vi "Nicmos_Diagnostics.vi"() -> ()   [LabVIEW 2009]
panel:
  in  "Difference:":bool
  out "Waveform at Coord":dbl[](graph)
  out "Intensity Map At Index":dbl[][](graph)
  in  "stop":bool
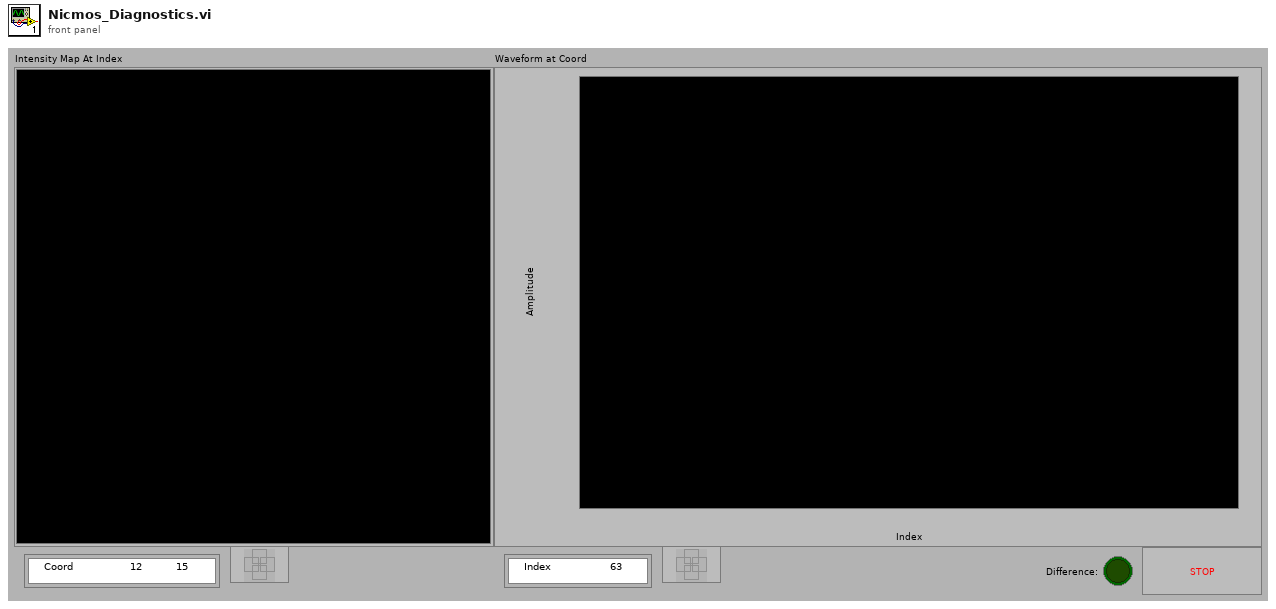
[diagram p1: front panel]
types:
  T1 = typedef "LVPointDoubleTypeDef.ctl" = cluster{"Cursor X":dbl, "Cursor Y":dbl}
  T2 = typedef "NICMOS.RAW.ctl" = u16[][][]
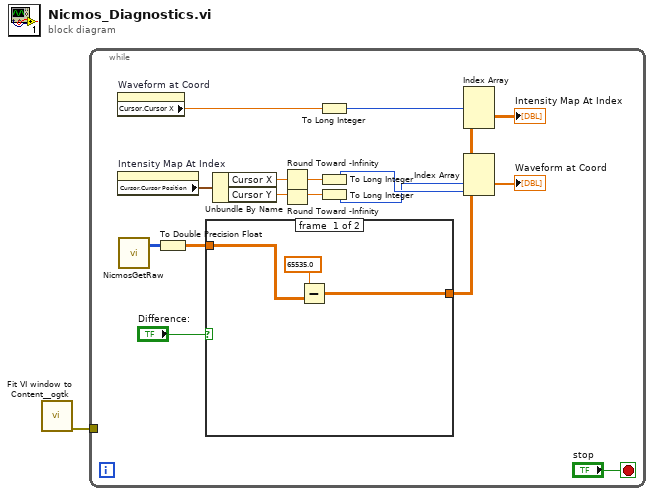
[diagram p0: block diagram]
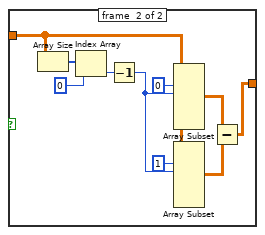
[diagram p2: hidden frame]
diagram:
  n1 = call <userlib>:"Fit VI window to Content__ogtk.vi"() -> ("error out"=w1:errorcluster)  [unwired: 6 in, 1 out]
  n2 = while {
    tunnel: w1 -> [_]
    stop <- "stop" stop-if-true
    n3 = property on="Waveform at Coord" class="WFGraph (strict)"() -> ("Cursor.Cursor X"=w8:dbl)  [unwired: 2 in, 2 out]
    n4 = property on="Intensity Map At Index" class="IntGraph (strict)"() -> ("Cursor.Cursor Position"=w13:T1)  [unwired: 2 in, 2 out]
    n5 = call "NicmosGetRaw.vi"() -> ("NICMOS.RAW"=w16:T2)  [unwired: 8 in, 1 out]
    n6 = To Double Precision Float(number=w16) -> (double precision float=w4:dbl[][][])
    n7 = case shown="True" "Difference:" {
      tunnel: w4 -> [w20 w28]
      tunnel: [w19 w21] -> w3
      frame #0 {
        n8 = Subtract(x=65535.0, y=w20) -> (x-y=w19:dbl[][][])
      }
      frame #1 {
        n9 = Array Size(array=w28) -> (size(s)=w27:i32[])
        n10 = Index Array(array=w27, index=0) -> (element=w25:i32)
        n11 = Decrement(x=w25) -> (x-1=w24:i32)
        n12 = Array Subset(array=w28, index (dim 0)=0 ("index"), length (dim 0)=w24) -> (w23:dbl[][][])  [unwired: 4 in]
        n13 = Array Subset(array=w28, index (dim 0)=1 ("index"), length (dim 0)=w24) -> (w22:dbl[][][])  [unwired: 4 in]
        n14 = Subtract(x=w23, y=w22) -> (x-y=w21:dbl[][][])
      }
    }
    n15 = Unbundle By Name(w13) -> ("Cursor X"=w12:dbl, "Cursor Y"=w11:dbl)
    n16 = Round Toward -Infinity(1:w12) -> (0:w6:dbl)
    n17 = Round Toward -Infinity(1:w11) -> (0:w5:dbl)
    n18 = To Long Integer(number=w8) -> (32bit integer=w7:i32)
    n19 = To Long Integer(number=w6) -> (32bit integer=w10:i32)
    n20 = To Long Integer(number=w5) -> (32bit integer=w9:i32)
    n21 = Index Array(array=w3, index (dim 0)=w7) -> (element=→"Intensity Map At Index":dbl[][])  [unwired: 2 in]
    n22 = Index Array(array=w3, index (dim 1)=w9, index (dim 2)=w10) -> (element=→"Waveform at Coord":dbl[])  [unwired: 1 in]
  }
